vi "database_password_prompt.vi"(8 "error_in":errorcluster) -> (0 "error_out":errorcluster, 2 "Canceled?":bool, 3 "new_password":string)   [LabVIEW 2020]
uses:
  AULocalize/SubVIs/RegisterVI.vi
  AULocalize/SubVIs/Get Localized Phrase Compact Interface 0D.vi
panel:
  out "prompt_info":string
  in  "Password:":string
  in  "Cancel":bool
  in  "OK":bool
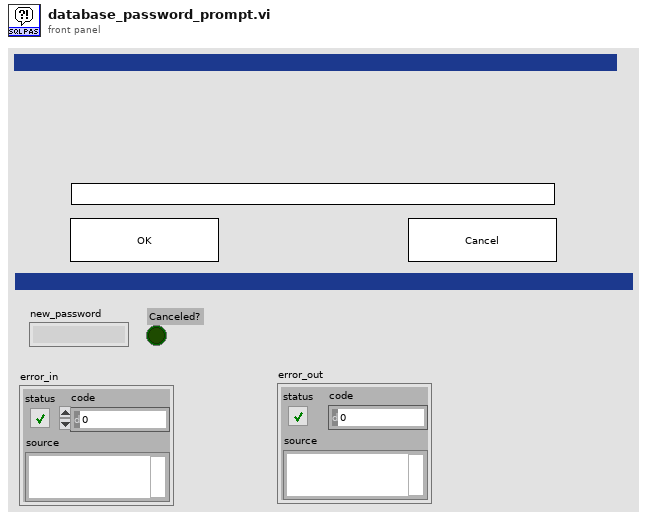
[diagram p1: front panel]
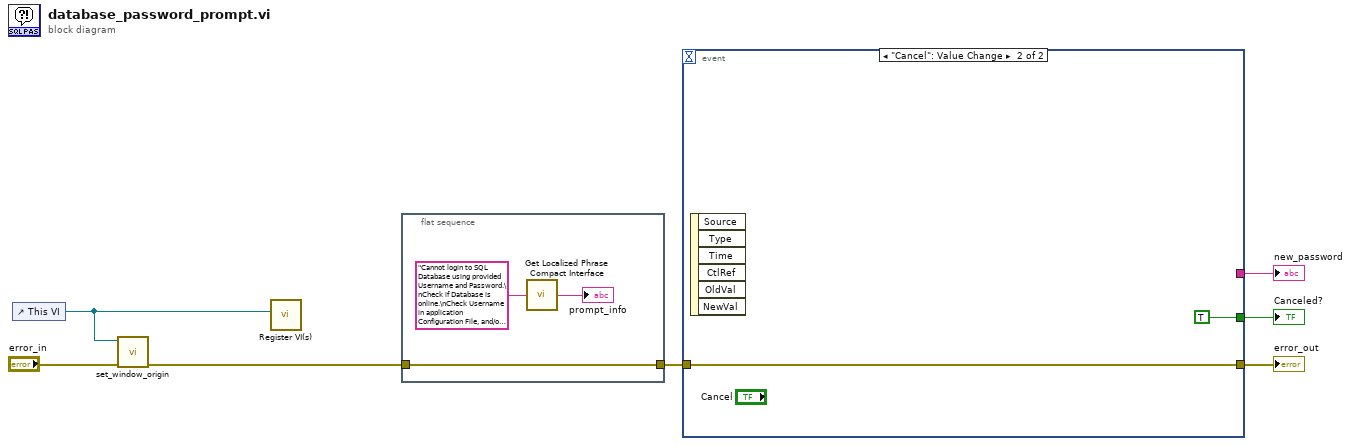
[diagram p0: block diagram]
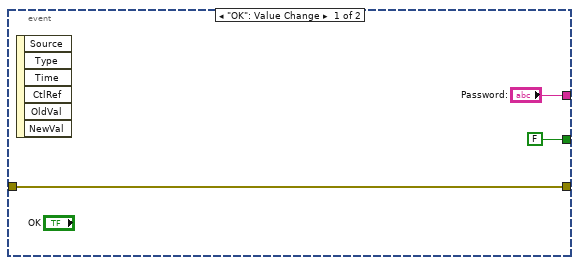
[diagram p2: hidden frame]
diagram:
  n1 = control-ref of="This VI"() -> (w2:refnum<vi>)
  n2 = call "set_window_origin.vi"("error_in"="error_in", "this_vi_reference"=w2) -> ("error_out"=w1:errorcluster)  [unwired: 9 in]
  n3 = call-poly "Register VI(s).vi"("VI Ref"=w2) -> ()  [unwired: 9 in, 2 out]
  n4 = flat-sequence {
    tunnel: w1 -> [w8]
    tunnel: [w8] -> w3
    frame #0 {
      n5 = call-poly "Get Localized Phrase Compact Interface.vi"("Key"="Cannot login to SQL Database using provided Username and Password.\nCheck if Database is online.\nCheck Username in application Configuration File, and/or enter correct\nPassword in the field below:") -> ("Translated Phrase"=→"prompt_info":string)
    }
  }
  n6 = event shown="[1] \"Cancel\": Value Change" {
    selector: _ -> [_ _]
    dyn-events: _ -> [_ _]
    timeout: _ -> [_ _]
    tunnel: [FALSE TRUE] -> w7
    tunnel: w3 -> [w12 w14]
    tunnel: [w12 w14] -> w5
    tunnel: ["Password:" _] -> w4
    event "OK": Value Change {
      n7 = event-data() -> ()  [unwired: 1 in, 6 out]
    }
    event "Cancel": Value Change {
      n8 = event-data() -> ()  [unwired: 1 in, 6 out]
    }
  }
  "Canceled?" <- w7
  "error_out" <- w5
  "new_password" <- w4
